vi "get_commit_hash.vi"(6 "quiet?":bool=TRUE, 8 "error in (no error)":errorcluster, 11 "path":path) -> (0 "error out":errorcluster, 3 "commit_hash":string)   [LabVIEW 2015, in "lv-bin-git.lvlib" / "v1.lvlib"]
uses:
  v1.lvlib
  <userlib>/antonio-alexander/lv-bin/lv-bin/public/api/v1/v1.lvlib
  lv-bin-git.lvlib
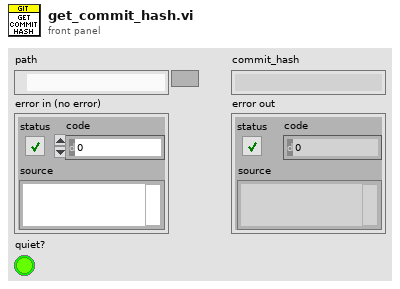
[diagram p1: front panel]
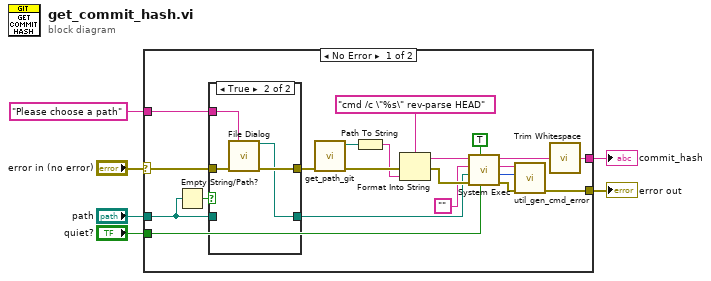
[diagram p0: block diagram]
diagram:
  n1 = case shown="No Error" "error in (no error)" {
    selector: "error in (no error)" -> [w23 w34]
    tunnel: [w17 w34] -> w2
    tunnel: "path" -> [w22 _]
    tunnel: "Please choose a path" ("prompt") -> [w20 _]
    tunnel: "quiet?" -> [w16 _]
    tunnel: [w7 _] -> w3
    frame No Error {
      n2 = Empty String/Path?(string/path=w22) -> (empty?=w21:bool)
      n3 = case shown="True" w21 {
        tunnel: w23 -> [w28 w33]
        tunnel: [w28 w32] -> w11
        tunnel: w22 -> [w29 _]
        tunnel: w20 -> [_ w31]
        tunnel: [w29 w30] -> w8
        frame False {
        }
        frame True {
          n4 = call "File Dialog"("prompt"=w31, "error in"=w33) -> ("selected path"=w30:path, "error out"=w32:errorcluster)  [unwired: 10 in, 2 out]
        }
      }
      n5 = call "get_path_git.vi"("error in (no error)"=w11) -> ("error out"=w12:errorcluster, "git.exe"=w10:path)  [unwired: 9 in]
      n6 = Path To String(path=w10) -> (string=w9:string)
      n7 = Format Into String(format string="cmd /c \"%s\" rev-parse HEAD", error in=w12, w9) -> (resulting string=w26:string, error out=w27:errorcluster)  [unwired: 1 in]
      n8 = call <vilib>:"System Exec.vi"("run minimized? (F)"=w16, "wait until completion? (T)"=TRUE, "error in (no error)"=w27, "working directory"=w8, "standard input"="", "command line"=w26) -> ("error out"=w18:errorcluster, "return code"=w13:i32, "standard error"=w15:string, "standard output"=w14:string)  [unwired: 2 in]
      n9 = call <userlib>:"util_gen_cmd_error.vi"("error in (no error)"=w18, "return_code"=w13, "standard_error"=w15) -> ("error out"=w17:errorcluster)  [unwired: 8 in]
      n10 = call <vilib>:"Trim Whitespace.vi"("string"=w14) -> ("trimmed string"=w7:string)  [unwired: 1 in]
    }
    frame Error {
    }
  }
  "error out" <- w2
  "commit_hash" <- w3
